vi "SelectSimulationParameter.vi"(5 "Day of Year":u32, 7 "Day Time":u32, 8 "error in (no error)":errorcluster, 9 "Type of Simulation":u16(ring) items=["External Network", "Consumer", "Producer", "Sorage"], 10 "Unique Object Identifier":string, 11 "SimulationParameter in":refnum<class "SimulationParameter.lvclass">) -> (0 "error out":errorcluster, 2 "Cluster":T1, 3 "SimulationParameter out":refnum<class "SimulationParameter.lvclass">)   [LabVIEW 2017, in "SimulationParameter.lvclass"]
uses:
  SimulationParameter.lvclass
  SimulationParameter.lvclass/SimulationParameter.ctl
  <vilib>/drjdpowell/SQLite Library/SQL Statement/SQL Statement.lvclass/SQL Statement.ctl
  <vilib>/drjdpowell/SQLite Library/SQL Statement/Column DBL.vi
  <vilib>/drjdpowell/SQLite Library/SQL Statement/Column I64.vi
  <vilib>/drjdpowell/SQLite Library/SQL Statement/Step.vi
  <vilib>/drjdpowell/SQLite Library/SQL Statement/Column Type.vi
  <vilib>/drjdpowell/SQLite Library/SQL Statement/Error Message.vi
  <vilib>/drjdpowell/SQLite Library/SQL Statement/Column String.vi
  <vilib>/drjdpowell/SQLite Library/SQL Statement/SQL Statement.lvclass
  <vilib>/drjdpowell/SQLite Library/SQL Connection/Connection.lvclass
panel:
  # "1 - 'Operating Timetable', \n2 - 'El. Energy In',  \n3 - 'El. Energy Out', \n4 - 'Th. Energy In',  \n5 - 'Th. Energy Out',  \n6 - 'Maximum el. Power', \n7 - 'Minimal el. Power', \n8 - 'Maximum th. Power', \n9 - 'Minimal th. Power', \n10 - 'El. Capacity',  \n11 - 'Th. Capacity',\n12 - 'El. Charge State at Start', \n13 - 'Th. Charge State at Start', \n14 - 'Activity (on / off) at Start',"
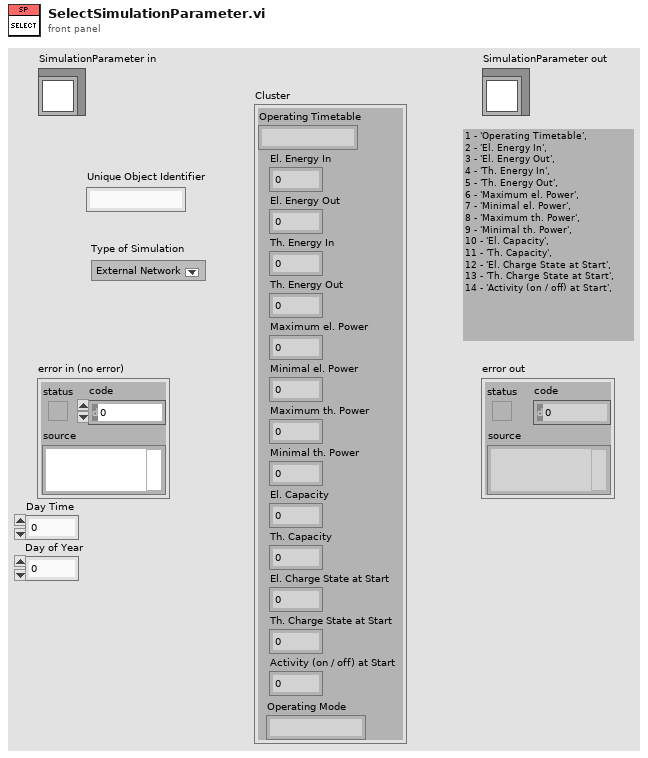
[diagram p1: front panel]
types:
  T1 = cluster{"Operating Timetable":string, "El. Energy In":dbl, "El. Energy Out":dbl, "Th. Energy In":dbl, "Th. Energy Out":dbl, "Maximum el. Power":dbl, "Minimal el. Power":dbl, "Maximum th. Power":dbl, "Minimal th. Power":dbl, "El. Capacity":dbl, "Th. Capacity":dbl, "El. Charge State at Start":dbl, "Th. Charge State at Start":dbl, "Activity (on / off) at Start":i64, "Operating Mode":string}
  T2 = cluster{"Column:Get Column String":string, "Column:Get Column DBL":dbl, "Column:Get Column DBL":dbl, "Column:Get Column DBL":dbl, "Column:Get Column DBL":dbl, "Column:Get Column DBL":dbl, "Column:Get Column DBL":dbl, "Column:Get Column DBL":dbl, "Column:Get Column DBL":dbl, "Column:Get Column DBL":dbl, "Column:Get Column DBL":dbl, "Column:Get Column DBL":dbl, "Column:Get Column DBL":dbl, "Column:Get Column I64":i64, "Column:Get Column String":string}
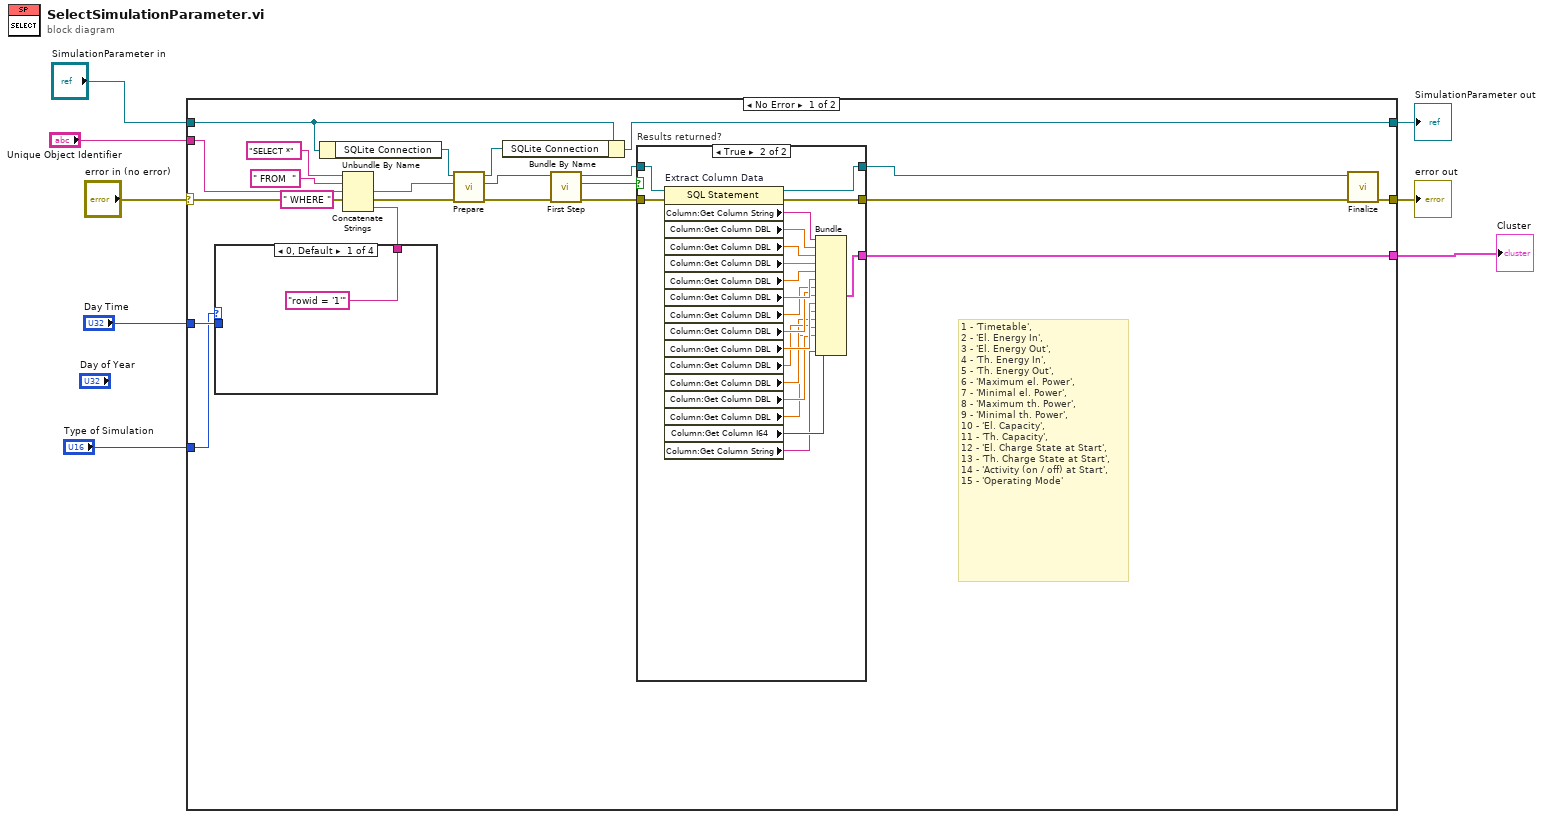
[diagram p0: block diagram]
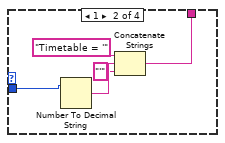
[diagram p2: hidden frame]
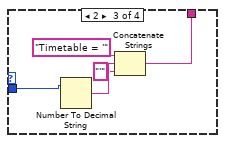
[diagram p3: hidden frame]
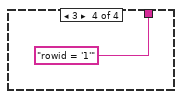
[diagram p4: hidden frame]
diagram:
  n1 = case shown="No Error" "error in (no error)" {
    selector: "error in (no error)" -> [w19 w66]
    tunnel: [w18 w66] -> w4
    tunnel: [w21 w65] -> w6
    tunnel: "SimulationParameter in" -> [w22 w65]
    tunnel: "Unique Object Identifier" -> [w16 _]
    tunnel: [w14 _] -> w3
    tunnel: "Day Time" -> [w11 _]
    tunnel: "Type of Simulation" -> [w9 _]
    frame No Error {
      # "1 - 'Timetable', \n2 - 'El. Energy In',  \n3 - 'El. Energy Out', \n4 - 'Th. Energy In',  \n5 - 'Th. Energy Out',  \n6 - 'Maximum el. Power', \n7 - 'Minimal el. Power', \n8 - 'Maximum th. Power', \n9 - 'Minimal th. Power', \n10 - 'El. Capacity',  \n11 - 'Th. Capacity',\n12 - 'El. Charge State at Start', \n13 - 'Th. Charge State at Start', \n14 - 'Activity (on / off) at Start',\n15 - 'Operating Mode'"
      n2 = case shown="0, Default" w9 {
        tunnel: w11 -> [_ w36 w41 _]
        tunnel: ["rowid = '1'" w35 w40 "rowid = '1'"] -> w10
        frame 0, Default {
        }
        frame 1 {
          n3 = Number To Decimal String(number=w36) -> (decimal integer string=w33:string)  [unwired: 1 in]
          n4 = Concatenate Strings("Timetable = '", w33, "'" ("string")) -> (w35:string)
        }
        frame 2 {
          n5 = Number To Decimal String(number=w41) -> (decimal integer string=w38:string)  [unwired: 1 in]
          n6 = Concatenate Strings("Timetable = '", w38, "'" ("string")) -> (w40:string)
        }
        frame 3 {
        }
      }
      n7 = Unbundle By Name(w22) -> ("SQLite Connection"=w23:refnum<class "Connection.lvclass">)
      n8 = Concatenate Strings("SELECT *" ("string"), " FROM  " ("string"), w16, " WHERE " ("string"), w10) -> (w15:string)
      n9 = call <vilib>:"Prepare.vi"("error in (no error)"=w19, "SQL"=w15, "SQLite Connection in"=w23) -> ("error out"=w24:errorcluster, "SQL Statement out"=w25:refnum<class "SQL Statement.lvclass">, "SQLite Connection out"=w20:refnum<class "Connection.lvclass">)  [unwired: 4 in, 2 out]
      n10 = Bundle By Name(cluster=w22, "SQLite Connection"=w20) -> (w21:refnum<class "SimulationParameter.lvclass">)
      n11 = call <vilib>:"First Step.vi"("error in (no error)"=w24, "SQL Statement in"=w25) -> ("error out"=w27:errorcluster, "Row returned"=w26:bool, "SQL Statement out"=w28:refnum<class "SQL Statement.lvclass">)  [unwired: 7 in]
      n12 = case "Results returned?" shown="True" w26 {
        tunnel: [w44 w61] -> w29
        tunnel: [w43 w62] -> w30
        tunnel: w28 -> [w44 w64]
        tunnel: w27 -> [w43 w63]
        tunnel: [_ w56] -> w14
        frame False {
        }
        frame True {
          n13 = property on="Extract Column Data" class="SQL Statement"(reference=w64, error in=w63) -> (reference out=w61:refnum<class "SQL Statement.lvclass">, error out=w62:errorcluster, "Column:Get Column String"=w60:string, "Column:Get Column DBL"=w59:dbl, "Column:Get Column DBL"=w58:dbl, "Column:Get Column DBL"=w55:dbl, "Column:Get Column DBL"=w57:dbl, "Column:Get Column DBL"=w54:dbl, "Column:Get Column DBL"=w53:dbl, "Column:Get Column DBL"=w52:dbl, "Column:Get Column DBL"=w51:dbl, "Column:Get Column DBL"=w50:dbl, "Column:Get Column DBL"=w49:dbl, "Column:Get Column DBL"=w48:dbl, "Column:Get Column DBL"=w47:dbl, "Column:Get Column I64"=w46:i64, "Column:Get Column String"=w45:string)
          n14 = Bundle("Column:Get Column String"=w60, "Column:Get Column DBL"=w59, "Column:Get Column DBL"=w58, "Column:Get Column DBL"=w55, "Column:Get Column DBL"=w57, "Column:Get Column DBL"=w54, "Column:Get Column DBL"=w53, "Column:Get Column DBL"=w52, "Column:Get Column DBL"=w51, "Column:Get Column DBL"=w50, "Column:Get Column DBL"=w49, "Column:Get Column DBL"=w48, "Column:Get Column DBL"=w47, "Column:Get Column I64"=w46, "Column:Get Column String"=w45) -> (w56:T2)  [unwired: 1 in]
        }
      }
      n15 = call <vilib>:"Finalize.vi"("error in (no error)"=w30, "SQL Statement in"=w29) -> ("error out"=w18:errorcluster)  [unwired: 9 in]
    }
    frame Error {
    }
  }
  "error out" <- w4
  "SimulationParameter out" <- w6
  "Cluster" <- w3
